vi "Task1.vi"() -> ()   [LabVIEW 2017]
panel:
  out "LED 8":bool
  out "LED 7":bool
  out "LED 6":bool
  out "LED 5":bool
  out "LED 4":bool
  out "LED 3":bool
  out "LED 2":bool
  in  "SW 8":bool
  in  "SW 7":bool
  in  "SW 6":bool
  in  "SW 5":bool
  in  "SW 4":bool
  in  "SW 3":bool
  in  "SW 2":bool
  out "LED 1":bool
  in  "SW 1":bool
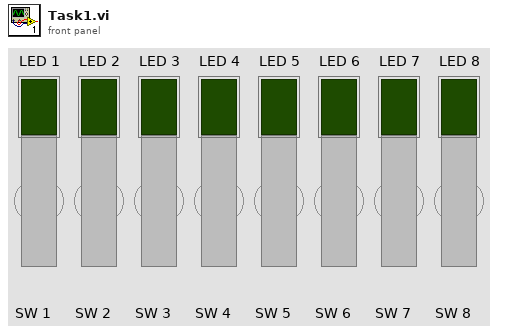
[diagram p1: front panel]
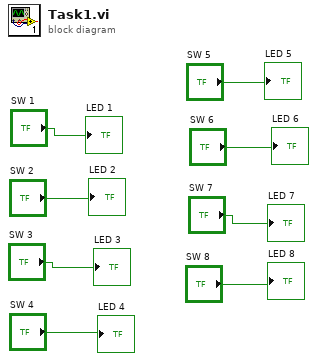
[diagram p0: block diagram]
diagram:
  "LED 1" <- "SW 1"
  "LED 2" <- "SW 2"
  "LED 3" <- "SW 3"
  "LED 4" <- "SW 4"
  "LED 5" <- "SW 5"
  "LED 6" <- "SW 6"
  "LED 7" <- "SW 7"
  "LED 8" <- "SW 8"
